vi "Get External Trigger Termination.vi"(11 "puiTermination":u32) -> (2 "function return":u32, 3 "puiTermination out":u32)   [LabVIEW 2018, in "Copy of Andor SDK.lvlib"]
doc: "EXPNETTYPE unsigned int WINAPI GetExternalTriggerTermination(at_u32 * puiTermination);"
uses:
  Copy of Andor SDK.lvlib
  <userlib>/Andor SDK/ATMCD32D.dll
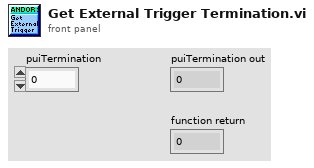
[diagram p1: front panel]
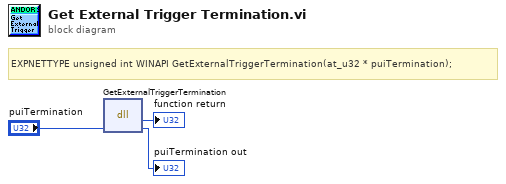
[diagram p0: block diagram]
diagram:
  # "EXPNETTYPE unsigned int WINAPI GetExternalTriggerTermination(at_u32 * puiTermination);"
  n1 = dll-call lib="C:/Program Files (x86)/National Instruments/LabVIEW 2018/user.lib/Andor SDK/ATMCD32D.*" fn="GetExternalTriggerTermination"("puiTermination"="puiTermination") -> (→"function return":u32, "puiTermination"=→"puiTermination out":u32)  [unwired: 3 in, 2 out]
